vi "Import Export - Temp SDF Create.vi"(8 "Error In":errorcluster, 11 "Item Ref in":T1 format="%.0x") -> (0 "Error Out":errorcluster, 1 "Temp SDF Path Out":path, 2 "Temp SDF Refnum":refnum<k24>, 3 "Item Ref out":T1 format="%.0x")   [LabVIEW 2017, in "Scan Engine Custom Device.lvlib"]
uses:
  Scan Engine Custom Device.lvlib
  <vilib>/NI Veristand/Custom Device API/Custom Device Item Ref.ctl
  NationalInstruments.VeriStand.SystemDefinitionAPI
  NationalInstruments.VeriStand.SystemStorage
  <vilib>/NI Veristand/Custom Device API/Custom Device API.lvlib
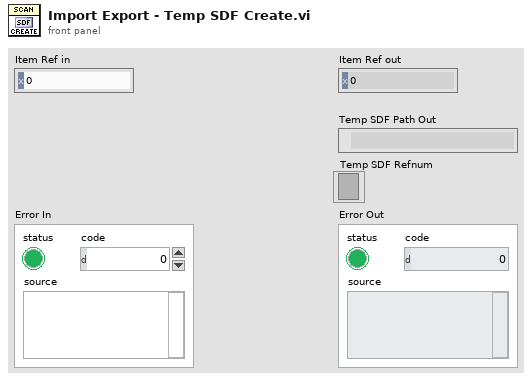
[diagram p1: front panel]
types:
  T1 = typedef "Custom Device API.lvlib/Custom Device Item Ref.ctl" = u64
  T2 = cluster{"Creator":string, "Description":string, "Target Name":string}
  T3 = typedef "Custom Device API.lvlib/Custom Device Pointer.ctl" = refnum<k24>
  T4 = typedef "Custom Device API.lvlib/Custom Device Target Type.ctl" = enum16{"PharLap", "VxWorks", "Windows", "Linux_32_ARM", "Linux_x64"}
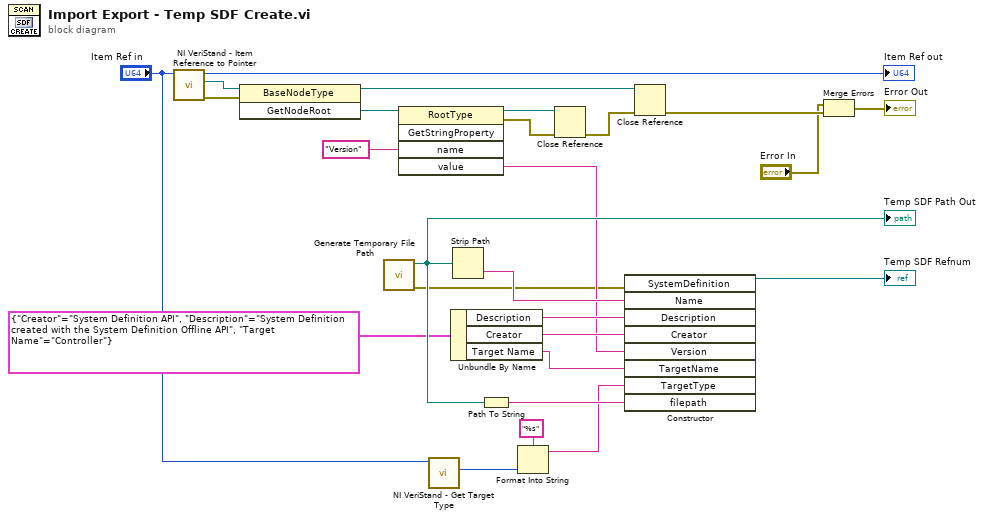
[diagram p0: block diagram]
diagram:
  n1 = call <vilib>:"NI VeriStand - Item Reference to Pointer.vi"("Item Ref in"="Item Ref in") -> ("error out"=w16:errorcluster, "Node Pointer"=w17:T3, "Item Ref out"=→"Item Ref out":T1)  [unwired: 7 in, 1 out]
  n2 = invoke class="BaseNodeType" method="GetNodeRoot"(reference=w17, error in=w16) -> (reference out=w13:T3, "GetNodeRoot"=w20:refnum<k24>)  [unwired: 1 in, 1 out]
  n3 = call <vilib>:"Generate Temporary File Path.vi"() -> ("error out"=w8:errorcluster, "Unique Temporary File Path"=w22:path)  [unwired: 10 in]
  "Temp SDF Path Out" <- w22
  n4 = invoke class="RootType" method="GetStringProperty"(reference=w20, "name"="Version") -> (reference out=w18:refnum<k24>, error out=w19:errorcluster, "value"=w10:string)  [unwired: 3 in, 2 out]
  n5 = call <vilib>:"NI VeriStand - Get Target Type.vi"("Item Ref in"="Item Ref in") -> ("Target Type"=w4:T4)  [unwired: 8 in, 2 out]
  n6 = Unbundle By Name(T2 {"Creator"="System Definition API", "Description"="System Definition created with the System Definition Offline API", "Target Name"="Controller"} ("New SDF Information")) -> ("Description"=w24:string, "Creator"=w25:string, "Target Name"=w3:string)
  n7 = Strip Path(path=w22) -> (name=w11:string)  [unwired: 1 out]
  n8 = Path To String(path=w22) -> (string=w26:string)
  n9 = Format Into String(format string="%s", w4) -> (resulting string=w2:string)  [unwired: 2 in, 1 out]
  n10 = Close Reference(reference=w18, error in (no error)=w19) -> (error out=w14:errorcluster)
  n11 = constructor class="SystemDefinition"(error in=w8, "Name"=w11, "Description"=w24, "Creator"=w25, "Version"=w10, "TargetName"=w3, "TargetType"=w2, "filepath"=w26) -> (reference out=→"Temp SDF Refnum":refnum<k24>)  [unwired: 2 in, 9 out]
  n12 = Close Reference(reference=w13, error in (no error)=w14) -> (error out=w9:errorcluster)
  n13 = Merge Errors("Error In", w9) -> (→"Error Out":errorcluster)
